vi "F Dwf Analog IO Channel Node Name.vi"(6 "szNodeUnits":string, 7 "szNodeName":string, 8 "error in (no error)":errorcluster, 9 "idxNode":i32, 10 "idxChannel":i32, 11 "hdwf":i32) -> (0 "error out":errorcluster, 3 "function return":i32, 4 "szNodeUnits out":string, 5 "szNodeName out":string)   [LabVIEW 2021, in "Olasdwf.lvlib"]
doc: "DWFAPI int FDwfAnalogIOChannelNodeName(HDWF hdwf, int idxChannel, int idxNode, char szNodeName[32], char szNodeUnits[16]);"
uses:
  Olasdwf.lvlib
  Windows/System32/dwf.dll
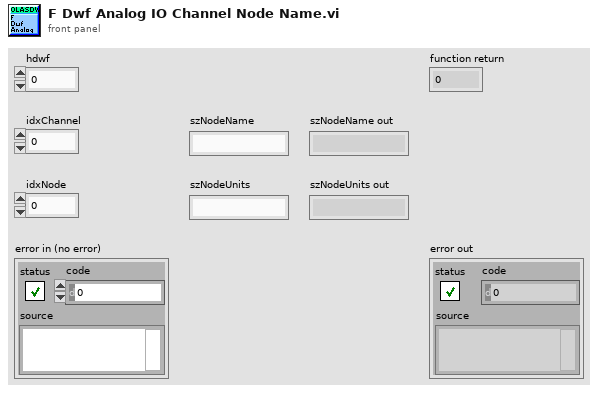
[diagram p1: front panel]
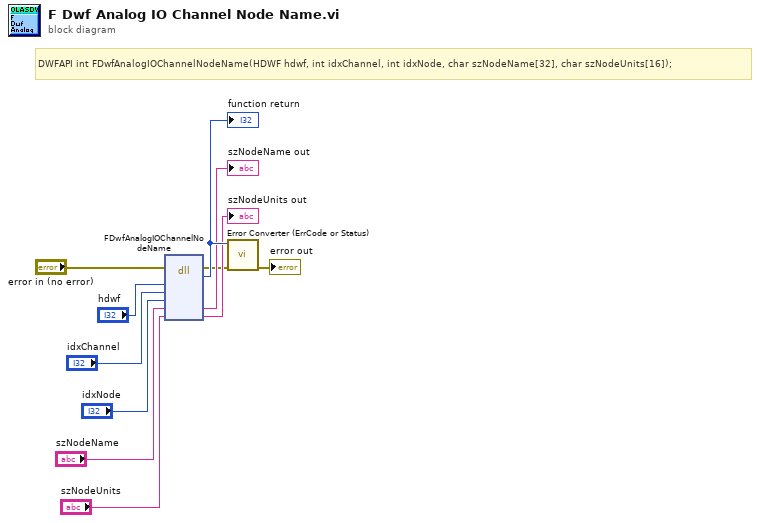
[diagram p0: block diagram]
diagram:
  # "DWFAPI int FDwfAnalogIOChannelNodeName(HDWF hdwf, int idxChannel, int idxNode, char szNodeName[32], char szNodeUnits[16]);"
  n1 = dll-call lib="/Windows/System32/dwf.*" fn="FDwfAnalogIOChannelNodeName"(error in="error in (no error)", "hdwf"="hdwf", "idxChannel"="idxChannel", "idxNode"="idxNode", "szNodeName"="szNodeName", "szNodeUnits"="szNodeUnits") -> (error out=w2:errorcluster, w11:i32, "szNodeName"=→"szNodeName out":string, "szNodeUnits"=→"szNodeUnits out":string)  [unwired: 5 in, 1 out]
  "function return" <- w11
  n2 = call "Error Converter (ErrCode or Status).vi"("error in (no error)"=w2, "error code"=w11) -> ("error out"=→"error out":errorcluster)  [unwired: 9 in]
